vi "Display_AE.vi"(7 "Action":enum16{"READ", "WRITE"}(ring), 10 "Display Array In":u8[][](array[numeric])) -> (2 "Display Array Out":u8[][](array[numeric]))   [LabVIEW 2014]
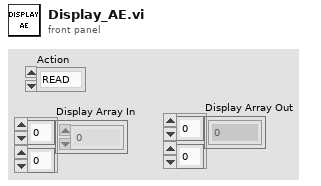
[diagram p1: front panel]
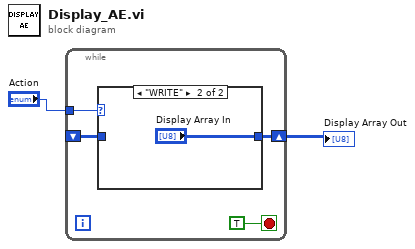
[diagram p0: block diagram]
diagram:
  n1 = while {
    shift-right: [w5] -> w2
    shift-left: _ -> [w3]
    tunnel: "Action" -> [w4]
    stop <- TRUE stop-if-true
    n2 = case shown="\"WRITE\"" w4 {
      tunnel: [w7 "Display Array In"] -> w5
      tunnel: w3 -> [w7 _]
      frame "READ", Default {
      }
      frame "WRITE" {
      }
    }
  }
  "Display Array Out" <- w2
